vi "Odd_Even.vi"() -> ()   [LabVIEW 2024]
uses:
  <vilib>/numeric/Random Number (Range) U64.vi
  <vilib>/numeric/sub_Random U32.vi
panel:
  out "Array 2":dbl[](array[numeric])
  out "Array":u64[](array[numeric])
  in  "Numeric":i32
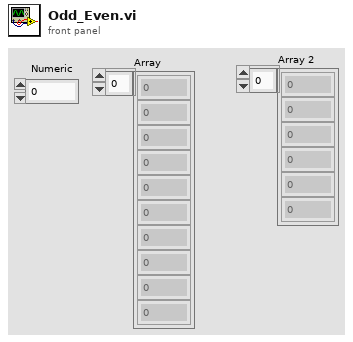
[diagram p1: front panel]
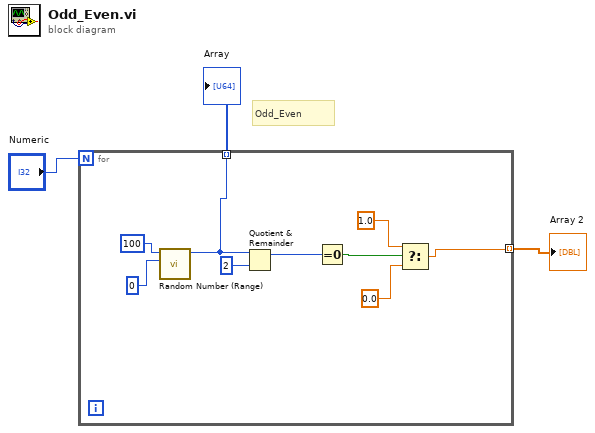
[diagram p0: block diagram]
diagram:
  # "Odd_Even"
  n1 = for {
    N: "Numeric" -> [_]
    tunnel: [w5] -> w2 mode=indexing
    tunnel: [w4] -> w1 mode=indexing
    n2 = call-poly <vilib>:"Random Number (Range).vi"("lower bound (0)"=u64 0, "upper bound (100)"=u64 100) -> ("number"=w5:u64)  [unwired: 9 in]
    n3 = Quotient & Remainder(x=w5, y=u64 2) -> (x-y*floor(x/y)=w11:u64)  [unwired: 1 out]
    n4 = Equal To 0?(x=w11) -> (x = 0?=w8:bool)
    n5 = Select(t=1.0, s=w8, f=0.0) -> (s? t:f=w4:dbl)
  }
  "Array" <- w2
  "Array 2" <- w1
